vi "CLD3 FGV Timer Solution.vi"(8 "Error In":errorcluster, 10 "Time Target (s)":dbl=4.0, 11 "Timer Mode":T1) -> (0 "Error Out":errorcluster, 2 "Has Time Elapsed":bool, 3 "Elapsed Time (s.ss)":dbl)   [LabVIEW 2020]
doc: "CLD 3 Exercise"
uses:
  CLD3 FGV Mode.ctl
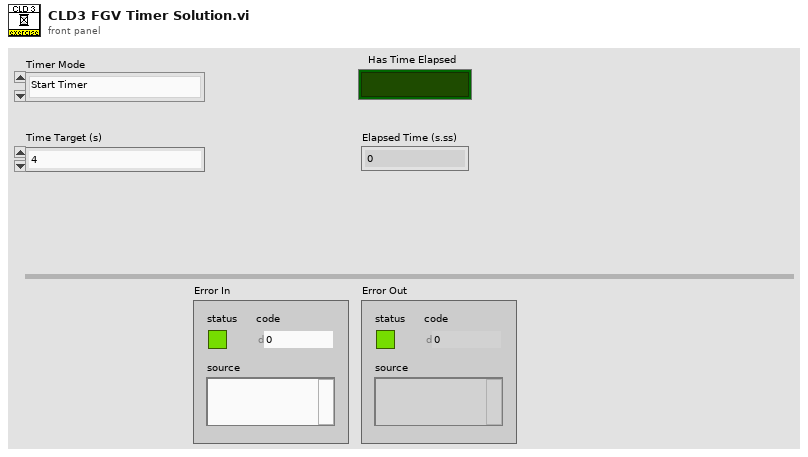
[diagram p1: front panel]
types:
  T1 = typedef "CLD3 FGV Mode.ctl" = enum16{"Start Timer", "Read Time", "Pause", "Resume"}
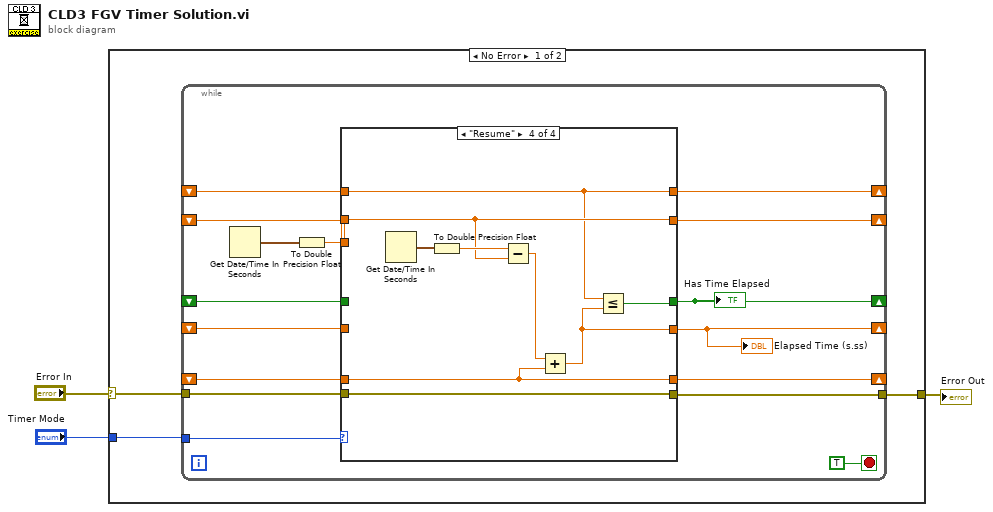
[diagram p0: block diagram]
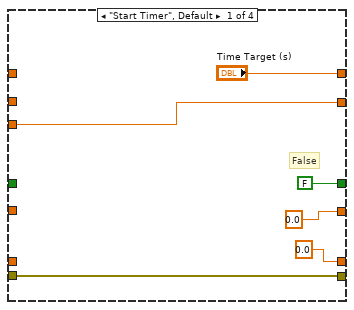
[diagram p2: hidden frame]
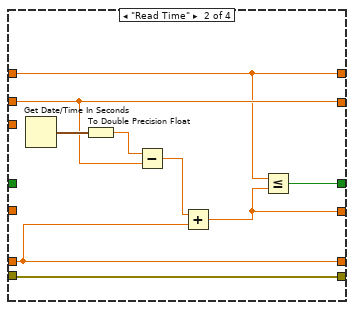
[diagram p3: hidden frame]
diagram:
  n1 = case shown="No Error" "Error In" {
    selector: "Error In" -> [w5 w52]
    tunnel: "Timer Mode" -> [w6 _]
    tunnel: [w4 w52] -> w1
    frame No Error {
      n2 = while {
        tunnel: w6 -> [w22]
        tunnel: w5 -> [w21]
        tunnel: [w20] -> w4
        shift-right: [w19] -> _
        shift-left: _ -> [w18]
        shift-right: [w17] -> _
        shift-left: _ -> [w16]
        shift-right: [w15] -> _
        shift-left: _ -> [w14]
        shift-right: [w11] -> _
        shift-left: _ -> [w8]
        shift-right: [w10] -> _
        shift-left: _ -> [w9]
        stop <- TRUE stop-if-true
        n3 = Get Date/Time In Seconds() -> (seconds since 1Jan1904=w13:timestamp)
        n4 = To Double Precision Float(number=w13) -> (double precision float=w12:dbl)
        n5 = case shown="\"Resume\"" w22 {
          tunnel: w21 -> [w28 w33 w42 w51]
          tunnel: [w28 w33 w42 w51] -> w20
          tunnel: ["Time Target (s)" w31 w41 w45] -> w19
          tunnel: w18 -> [_ w31 w41 w45]
          tunnel: [0.0 w30 w38 w44] -> w17
          tunnel: w16 -> [_ _ w38 _]
          tunnel: [FALSE w29 w39 w43] -> w15
          tunnel: w14 -> [_ _ w39 _]
          tunnel: w12 -> [w24 _ w40 _]
          tunnel: [w24 w34 w40 w48] -> w11
          tunnel: [0.0 w32 w38 w46] -> w10
          tunnel: w9 -> [_ w32 _ w46]
          tunnel: w8 -> [_ w34 _ w48]
          frame "Start Timer", Default {
            # "False"
          }
          frame "Read Time" {
            n6 = Get Date/Time In Seconds() -> (seconds since 1Jan1904=w37:timestamp)
            n7 = To Double Precision Float(number=w37) -> (double precision float=w36:dbl)
            n8 = Subtract(x=w36, y=w34) -> (x-y=w35:dbl)
            n9 = Add(x=w35, y=w32) -> (x+y=w30:dbl)
            n10 = Less Or Equal?(x=w31, y=w30) -> (x <= y?=w29:bool)
          }
          frame "Pause" {
          }
          frame "Resume" {
            n11 = Get Date/Time In Seconds() -> (seconds since 1Jan1904=w50:timestamp)
            n12 = To Double Precision Float(number=w50) -> (double precision float=w49:dbl)
            n13 = Subtract(x=w49, y=w48) -> (x-y=w47:dbl)
            n14 = Add(x=w47, y=w46) -> (x+y=w44:dbl)
            n15 = Less Or Equal?(x=w45, y=w44) -> (x <= y?=w43:bool)
          }
        }
        "Elapsed Time (s.ss)" <- w17
        "Has Time Elapsed" <- w15
      }
    }
    frame Error {
    }
  }
  "Error Out" <- w1
